vi "DriveList.vi"(9 "GL":bool=TRUE, 11 "Connection ID":T1) -> (2 "Drive":string[](array[string]), 3 "Connection ID Out":T1)   [LabVIEW 2017]
uses:
  Driver/ConnectionID.ctl
  GL860_Driver.lvlib
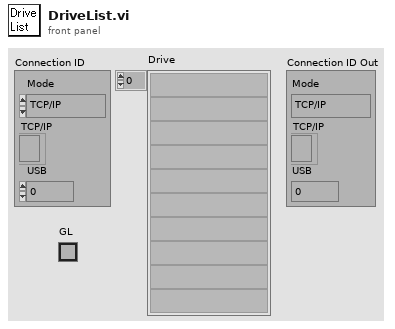
[diagram p1: front panel]
types:
  T1 = typedef "ConnectionID.ctl" = cluster{"Mode":enum16{"TCP/IP", "USB"}, "TCP/IP":refnum<k5>, "USB":i32}
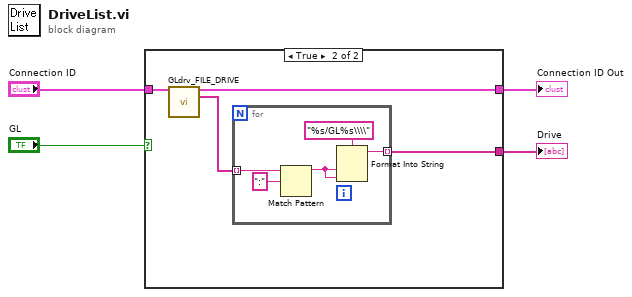
[diagram p0: block diagram]
diagram:
  n1 = case shown="TRUE" "GL" {
    tunnel: [w5 w9] -> w4
    tunnel: "Connection ID" -> [w5 w7]
    tunnel: [_ w6] -> w1
    frame False {
    }
    frame True {
      n2 = call "GLdrv_FILE_DRIVE.vi"("Connection ID"=w7) -> ("Connection ID Out"=w9:T1, "Drive out"=w8:string[])  [unwired: 12 in, 1 out]
      n3 = for {
        tunnel: w8 -> [w12] mode=indexing
        tunnel: [w13] -> w6 mode=indexing
        n4 = Match Pattern(string=w12, regular expression=":") -> (before substring=w11:string)  [unwired: 1 in, 3 out]
        n5 = Format Into String(format string="%s/GL%s\\\\", w11, w11) -> (resulting string=w13:string)  [unwired: 2 in, 1 out]
      }
    }
  }
  "Connection ID Out" <- w4
  "Drive" <- w1
